vi "HFRR ADV v033 new software.vi"() -> ()   [LabVIEW 2025] (continued)
            n2885 = call <vilib>:"Read Characters From File.vi"("file path (dialog if empty)"=w3937, "start of read offset (chars.:0)"=60 ("start of read offset (chars.: 0)")) -> ("character string"=→"String Indicator 2":string)  [unwired: 4 in, 3 out]
          }
        }
        n2886 = call <vilib>:"Query Available Printers.vi"() -> ("system configured printers"=w3629:string[])  [unwired: 9 in, 2 out]
        "System Configured Printers 2" <- w3629
        n2887 = local read "OK Button 16"() -> (w3626:bool)
        n2888 = case shown="True" "OK Button 16" {
          frame False {
          }
          frame True {
            n2889 = stacked-sequence {
              frame #0 {
                n2890 = local read "Numeric 16"() -> (w3954:i32)
                n2891 = local write "Numeric 10"(w3954) -> ()
              }
              frame #1 {
                n2892 = local read "String 29"() -> (w3957:string)
                n2893 = String To Path(string=w3957) -> (path=w3956:path)
                n2894 = Open/Create/Replace File "Open File"(file path (use dialog)=w3956) -> (refnum out=w3958:refnum<file>)  [unwired: 5 in, 2 out]
                n2895 = for {
                  N: 16 -> [_]
                  tunnel: w3958 -> [w3965]
                  i -> [w3961]
                  (unwired) TRUE ("line mode (F)")
                  n2896 = Read from Text File "Read File"(file (use dialog)=w3965) -> (text=w3959:string)  [unwired: 3 in, 3 out]
                  n2897 = Match Pattern(string=w3959, regular expression="(") -> (after substring=w3964:string)  [unwired: 1 in, 3 out]
                  n2898 = Match Pattern(string=w3964, regular expression=")") -> (before substring=w3960:string)  [unwired: 1 in, 3 out]
                  n2899 = case shown="1" w3961 {
                    tunnel: w3960 -> [w3966 w3967 _ _ w3968 w3969 w3970 w3972 w3974 w3976 w3978 w3980 w3982 w3984 _]
                    tunnel: w3959 -> [_ _ _ _ _ _ _ _ _ _ _ _ _ _ _]
                    frame 0 {
                      "TITTLE" <- w3966
                    }
                    frame 1 {
                      "Sample ID" <- w3967
                    }
                    frame 2 {
                    }
                    frame 3 {
                    }
                    frame 4 {
                      "Test Date" <- w3968
                    }
                    frame 5 {
                      "Tested by" <- w3969
                    }
                    frame 6 {
                      n2900 = Fract/Exp String To Number(string=w3970) -> (number=→"Humidity before test 2":dbl)  [unwired: 3 in, 1 out]
                    }
                    frame 7 {
                      n2901 = Fract/Exp String To Number(string=w3972) -> (number=→"Temperature before test 2":dbl)  [unwired: 3 in, 1 out]
                    }
                    frame 8 {
                      n2902 = Fract/Exp String To Number(string=w3974) -> (number=→"Humidity after test 2":dbl)  [unwired: 3 in, 1 out]
                    }
                    frame 9 {
                      n2903 = Fract/Exp String To Number(string=w3976) -> (number=→"Temperature after test 2":dbl)  [unwired: 3 in, 1 out]
                    }
                    frame 10 {
                      n2904 = Fract/Exp String To Number(string=w3978) -> (number=→"MWSD 2":dbl)  [unwired: 3 in, 1 out]
                    }
                    frame 11 {
                      n2905 = Fract/Exp String To Number(string=w3980) -> (number=→"AVP 2":dbl)  [unwired: 3 in, 1 out]
                    }
                    frame 12 {
                      n2906 = Fract/Exp String To Number(string=w3982) -> (number=→"HCF 2":dbl)  [unwired: 3 in, 1 out]
                    }
                    frame 13 {
                      n2907 = Fract/Exp String To Number(string=w3984) -> (number=→"WS1.4 2":dbl)  [unwired: 3 in, 1 out]
                    }
                    frame 14, Default {
                    }
                  }
                }
              }
              frame #2 {
              }
            }
            n2908 = local write "OK Button 16"(FALSE ("OK Button 13")) -> ()
          }
        }
        n2909 = Index Array(array=w3629, index="Select Printer 3") -> (element=w3631:string)
        "Selected Printer" <- w3631
        n2910 = case shown="True" w3626 {
          frame False {
          }
          frame True {
            n2911 = flat-sequence {
              frame #0 {
              }
              frame #1 {
                n2912 = Wait (ms)(milliseconds to wait=u32 100) -> ()  [unwired: 1 out]
              }
              frame #2 {
                n2913 = local write "OK Button 16"(FALSE ("Print 3")) -> ()
              }
            }
          }
        }
        n2914 = case shown="True" "Print" {
          tunnel: w3631 -> [_ w3923]
          frame False {
          }
          frame True {
            (unwired) i16 6 ("width (-)")
            (unwired) "TESTED BY : "
            (unwired) "TESTED DATE :"
            (unwired) "SAMPLE ID : "
            (unwired) "SAMPLE DESIGN : "
            w3881 = "\r"
            w3898 = "\r"
            # "add image"
            n2915 = local read "Sample ID"() -> (w3871:string)
            n2916 = local read "Tested by"() -> (w3874:string)
            n2917 = local read "String 34"() -> (w3861:string)
            n2918 = local read "String 45"() -> (w3841:string)
            n2919 = local read "String 35"() -> (w3856:string)
            n2920 = local read "String 37"() -> (w3854:string)
            n2921 = local read "String 32"() -> (w3876:string)
            n2922 = local read "String 36"() -> (w3851:string)
            n2923 = local read "String 31"() -> (w3875:string)
            n2924 = local read "Test Date"() -> (w3872:string)
            n2925 = local read "String 33"() -> (w3877:string)
            n2926 = local read "String 38"() -> (w3847:string)
            n2927 = local read "String 39"() -> (w3844:string)
            n2928 = local write "Print"(FALSE ("Print FF")) -> ()
            n2929 = local read "S 39"() -> (w3859:string)
            n2930 = local read "S 38"() -> (w3866:string)
            n2931 = local read "Temperature before test 2"() -> (w3897:dbl)
            n2932 = local read "Temperature after test 2"() -> (w3887:dbl)
            n2933 = local read "Humidity before test 2"() -> (w3912:dbl)
            n2934 = local read "Humidity after test 2"() -> (w3896:dbl)
            n2935 = local read "MWSD 2"() -> (w3901:dbl)
            n2936 = local read "WS1.4 2"() -> (w3879:dbl)
            n2937 = Concatenate Strings("2)" ("string"), w3861) -> (w3862:string)
            n2938 = Concatenate Strings("3)" ("string"), w3859) -> (w3860:string)
            n2939 = Concatenate Strings("1)" ("string"), w3866) -> (w3865:string)
            n2940 = Concatenate Strings("4)" ("string"), w3856) -> (w3857:string)
            n2941 = Concatenate Strings("5)" ("string"), w3854) -> (w3853:string)
            n2942 = Concatenate Strings("6)" ("string"), w3851) -> (w3850:string)
            n2943 = Concatenate Strings("7)" ("string"), w3847) -> (w3848:string)
            n2944 = Concatenate Strings("8)" ("string"), w3844) -> (w3845:string)
            n2945 = local read "HCF 2"() -> (w3883:dbl)
            n2946 = local read "AVP 2"() -> (w3900:dbl)
            n2947 = local read "s.NO"() -> (w3842:string)
            n2948 = call <vilib>:"New Report.vi"("report type"=enum16{"Standard Report", "HTML"}."Standard Report") -> ("report out"=w3921:refnum<class "NI_report.lvclass">, "error out"=w3920:errorcluster)  [unwired: 13 in]
            n2949 = local read "TITTLE"() -> (w3873:string)
            n2950 = Concatenate Strings(w3898, w3841, w3842, w3898, w3876, w3871, w3898, w3875, w3872, w3898, w3877, w3874, w3898) -> (w3891:string)
            "test by" <- w3891
            n2951 = Number To Fractional String(number=w3897, width (-)=i16 6, precision (6)=i16 2) -> (F-format string=w3886:string)  [unwired: 1 in]
            n2952 = Number To Fractional String(number=w3896, width (-)=i16 6, precision (6)=i16 2) -> (F-format string=w3899:string)  [unwired: 1 in]
            n2953 = Number To Fractional String(number=w3912, width (-)=i16 6, precision (6)=i16 2) -> (F-format string=w3917:string)  [unwired: 1 in]
            n2954 = Number To Fractional String(number=w3901, width (-)=i16 6, precision (6)=i16 2) -> (F-format string=w3903:string)  [unwired: 1 in]
            n2955 = Number To Fractional String(number=w3887, width (-)=i16 6, precision (6)=i16 2) -> (F-format string=w3888:string)  [unwired: 1 in]
            n2956 = Number To Fractional String(number=w3900, width (-)=i16 6, precision (6)=i16 2) -> (F-format string=w3902:string)  [unwired: 1 in]
            n2957 = Number To Fractional String(number=w3883, width (-)=i16 6, precision (6)=i16 2) -> (F-format string=w3882:string)  [unwired: 1 in]
            n2958 = Number To Fractional String(number=w3879, precision (6)=i16 2) -> (F-format string=w3878:string)  [unwired: 2 in]
            n2959 = call-dynamic "Set Report Header Text.vi"("report in"=w3921, "center header text"=w3873, "error in (no error)"=w3920) -> ("report out"=w3892:refnum<class "NI_report.lvclass">, "error out"=w3893:errorcluster)  [unwired: 11 in]
            n2960 = Concatenate Strings(w3881, w3865, w3917, w3881, w3862, w3886, w3881, w3860, w3899, w3881, w3857, w3888, w3881, w3853, w3903, w3881, w3850, w3902, w3881, w3848, w3882, w3881, w3845, w3878) -> (w3869:string)
            "export 2" <- w3869
            n2961 = call-poly <vilib>:"Append Report Text.vi"("report in"=w3892, "text"=w3891, "error in (no error)"=w3893) -> ("report out"=w3895:refnum<class "NI_report.lvclass">, "error out"=w3894:errorcluster)  [unwired: 9 in, 2 out]
            n2962 = local read "test by"() -> (w3868:string)
            n2963 = local read "TITTLE"() -> (w3870:string)
            n2964 = call-poly <vilib>:"Append Report Text.vi"("report in"=w3895, "error in (no error)"=w3894) -> ("report out"=w3916:refnum<class "NI_report.lvclass">, "error out"=w3914:errorcluster)  [unwired: 10 in, 2 out]
            n2965 = Concatenate Strings(w3870, w3869, w3868) -> (→"output":string)
            n2966 = call-poly <vilib>:"Append Report Text.vi"("report in"=w3916, "text"=w3869, "error in (no error)"=w3914) -> ("report out"=w3915:refnum<class "NI_report.lvclass">, "error out"=w3913:errorcluster)  [unwired: 9 in, 2 out]
            n2967 = call-dynamic "Print Report.vi"("report in"=w3915, "printer name (default)"=w3923, "error in (no error)"=w3913) -> ("report out"=w3925:refnum<class "NI_report.lvclass">, "error out"=w3926:errorcluster)  [unwired: 11 in]
            n2968 = call-dynamic "Dispose Report.vi"("report in"=w3925, "error in (no error)"=w3926) -> ()  [unwired: 13 in, 1 out]
          }
        }
        n2969 = case shown="True" "Print 2" {
          frame False {
          }
          frame True {
            n2970 = flat-sequence {
              frame #0 {
                n2971 = local read "s.NO"() -> (→"s.NO 2":string)
                n2972 = Wait (ms)(milliseconds to wait=u32 20) -> ()  [unwired: 1 out]
                n2973 = local read "Sample ID  3"() -> (→"Sample ID  6":string)
                n2974 = local read "Sample ID  4"() -> (→"Sample ID  7":string)
                n2975 = local read "Sample ID"() -> (→"Sample ID  2":string)
                n2976 = local read "Tested by"() -> (→"Tested by 2":string)
                n2977 = local read "Test Date"() -> (→"Test Date 2":string)
                n2978 = local read "Humidity after test 3"() -> (→"Humidity after test 4":dbl)
                n2979 = local read "Ref A Test Date :"() -> (→"TITTLE 4":string)
                n2980 = local read "Temperature before test 3"() -> (w3748:dbl)
                n2981 = local read "Temperature before test 3"() -> (→"Temperature after test 5":dbl)
                n2982 = local read "Temperature after test 3"() -> (→"Temperature after test 4":dbl)
                n2983 = local read "Humidity before test 3"() -> (→"Humidity before test 4":dbl)
                n2984 = local write "Temperature before test 3"(w3748) -> ()
                n2985 = local read "image data"() -> (w3739:T16)
                n2986 = String To Path(string="C:\\LAB-IQ\\im\\Temp_resized.jpg") -> (path=w3740:path)
                "path 2" <- w3740
                n2987 = call <vilib>:"Write JPEG File.vi"("image data"=w3739, "path to JPEG file"=w3740) -> ()  [unwired: 8 in, 2 out]
                "Ref A Test Date :" <- "Ref A Test Date :"
                "Ref B Test Date :" <- "Ref B Test Date :"
                "Ref B Scar Value :" <- "Ref B Scar Value :"
                "Ref A Scar Value :" <- "Ref A Scar Value :"
              }
              frame #1 {
                (unwired) HTML_Report_Image_Alignment."MIDDLE" ("alignment (default)")
                w3776 = u16 0 items=["portrait", "landscape"] ("orientation (portrait)")
                (unwired) HTML_Report_Image_Alignment."ABSMIDDLE" ("alignment (default)")
                (unwired) "TESTED BY : "
                (unwired) "TESTED DATE :"
                (unwired) "SAMPLE ID : "
                (unwired) "SAMPLE DESIGN : "
                w3809 = "\r"
                # "add image"
                n2988 = Wait (ms)(milliseconds to wait=u32 20) -> ()  [unwired: 1 out]
                n2989 = local read "Sample ID  2"() -> (w3802:string)
                n2990 = local read "Wear Scar X"() -> (w3774:dbl)
                "Length ( microns ) 2" <- w3774
                n2991 = local read "Wear Scar Y"() -> (w3773:dbl)
                "Wear Scar Y ( microns ) :" <- w3773
                n2992 = local read "Test Date 2"() -> (w3803:string)
                n2993 = local read "Tested by 2"() -> (w3804:string)
                n2994 = local read "String 46"() -> (w3800:string)
                n2995 = local read "String 48"() -> (w3806:string)
                n2996 = local read "String 47"() -> (w3805:string)
                n2997 = local read "String 49"() -> (w3807:string)
                n2998 = local read "String 10"() -> (w3760:string)
                n2999 = local read "s.NO 2"() -> (w3801:string)
                n3000 = Add(x=w3774, y=w3773) -> (x+y=w3772:dbl)
                n3001 = call <vilib>:"New Report.vi"("report type"=enum16{"Standard Report", "HTML"}."HTML") -> ("report out"=w3780:refnum<class "NI_report.lvclass">, "error out"=w3778:errorcluster)  [unwired: 13 in]
                n3002 = Concatenate Strings(w3809, w3800, w3801, w3809, w3806, w3802, w3809, w3805, w3803, w3809, w3807, w3804, w3809) -> (→"test by 2":string)
                n3003 = Concatenate Strings("C:\\LAB-IQ\\Data\\" ("string"), w3760, ".jpg" ("string")) -> ()  [unwired: 1 out]
                n3004 = Divide(x=w3772, y=2.0) -> (x/y=→"Mean Wear ( microns) :":dbl)
                n3005 = call-dynamic "Set Report Orientation.vi"("report in"=w3780, "orientation (portrait)"=w3776, "error in (no error)"=w3778) -> ("report out"=w3779:refnum<class "NI_report.lvclass">, "error out"=w3777:errorcluster)  [unwired: 11 in]
                n3006 = for {
                  N: 5 -> [_]
                  tunnel: w3779 -> [w3830]
                  tunnel: [w3829] -> w3758
                  tunnel: w3777 -> [w3828]
                  tunnel: [w3827] -> w3757
                  n3007 = call-dynamic "Set Report Tab Width.vi"("report in"=w3830, "error in (no error)"=w3828) -> ("report out"=w3829:refnum<class "NI_report.lvclass">, "error out"=w3827:errorcluster)  [unwired: 12 in]
                }
                n3008 = local read "TITTLE"() -> (w3775:string)
                n3009 = call-dynamic "Set Report Header Text.vi"("report in"=w3758, "center header text"=w3775, "error in (no error)"=w3757) -> ("report out"=w3796:refnum<class "NI_report.lvclass">, "error out"=w3795:errorcluster)  [unwired: 11 in]
                n3010 = for {
                  N: 1 -> [_]
                  tunnel: [w3834] -> w3782
                  tunnel: [w3833] -> w3781
                  tunnel: w3796 -> [w3832]
                  tunnel: w3795 -> [w3831]
                  n3011 = call-dynamic "New Report Line.vi"("report in"=w3832, "error in (no error)"=w3831) -> ("report out"=w3834:refnum<class "NI_report.lvclass">, "error out"=w3833:errorcluster)  [unwired: 12 in]
                }
                n3012 = for {
                  N: 2 -> [_]
                  tunnel: [w3826] -> w3788
                  tunnel: [w3825] -> w3787
                  tunnel: w3782 -> [w3824]
                  tunnel: w3781 -> [w3823]
                  n3013 = call-dynamic "New Report Line.vi"("report in"=w3824, "error in (no error)"=w3823) -> ("report out"=w3826:refnum<class "NI_report.lvclass">, "error out"=w3825:errorcluster)  [unwired: 12 in]
                }
                n3014 = for {
                  N: 25 -> [_]
                  tunnel: w3788 -> [w3822]
                  tunnel: w3787 -> [w3820]
                  tunnel: [w3821] -> w3791
                  tunnel: [w3819] -> w3790
                  n3015 = call-dynamic "Set Report Tab Width.vi"("report in"=w3822, "error in (no error)"=w3820) -> ("report out"=w3821:refnum<class "NI_report.lvclass">, "error out"=w3819:errorcluster)  [unwired: 12 in]
                }
                n3016 = control-ref of="Tab Control 9"() -> (w3786:refnum<vi>)
                n3017 = call-dynamic "Append Control Image to Report.vi"("report in"=w3791, "alignment (default)"=HTML_Report_Image_Alignment."ABSMIDDLE", "ctrl reference"=w3786, "error in (no error)"=w3790) -> ("report out"=w3785:refnum<class "NI_report.lvclass">, "error out"=w3784:errorcluster)  [unwired: 8 in, 2 out]
                n3018 = for {
                  N: 3 -> [_]
                  tunnel: [w3818] -> w3769
                  tunnel: [w3817] -> w3768
                  tunnel: w3785 -> [w3816]
                  tunnel: w3784 -> [w3815]
                  n3019 = call-dynamic "New Report Line.vi"("report in"=w3816, "error in (no error)"=w3815) -> ("report out"=w3818:refnum<class "NI_report.lvclass">, "error out"=w3817:errorcluster)  [unwired: 12 in]
                }
                n3020 = for {
                  N: 100 -> [_]
                  tunnel: w3769 -> [w3814]
                  tunnel: w3768 -> [w3812]
                  tunnel: [w3813] -> w3765
                  tunnel: [w3811] -> w3763
                  n3021 = call-dynamic "Set Report Tab Width.vi"("report in"=w3814, "error in (no error)"=w3812) -> ("report out"=w3813:refnum<class "NI_report.lvclass">, "error out"=w3811:errorcluster)  [unwired: 12 in]
                }
                n3022 = String To Path(string="C:\\LAB-IQ\\im\\Temp_resized.jpg") -> (path=w3755:path)
                n3023 = call-poly <vilib>:"Append Image to Report.vi"("report in"=w3765, "path or URL of image"=w3755, "error in (no error)"=w3763) -> ("report out"=w3764:refnum<class "NI_report.lvclass">, "error out"=w3762:errorcluster)  [unwired: 9 in, 2 out]
                n3024 = call-poly <vilib>:"Open HTML Report in Browser.vi"("report in"=w3764, "error in (no error)"=w3762) -> ("report out"=w3799:refnum<class "NI_report.lvclass">, "error out"=w3798:errorcluster)  [unwired: 11 in, 1 out]
                n3025 = call-dynamic "Dispose Report.vi"("report in"=w3799, "error in (no error)"=w3798) -> ()  [unwired: 13 in, 1 out]
              }
              frame #2 {
              }
              frame #3 {
                n3026 = disable-structure shown="Disabled" {
                  frame Disabled {
                    n3027 = local read "String 10"() -> (w3839:string)
                    n3028 = Concatenate Strings("C:\\LAB-IQ-NXT\\Data\\" ("string"), w3839, ".jpg" ("string")) -> (w3837:string)
                    n3029 = String To Path(string=w3837) -> (path=w3836:path)
                    n3030 = Delete(path (use dialog)=w3836) -> ()  [unwired: 4 in, 3 out]
                  }
                  frame Enabled {
                  }
                }
                n3031 = local write "Print 2"(FALSE ("Print")) -> ()
              }
            }
          }
        }
      }
    }
    n3032 = Wait (ms)(milliseconds to wait=u32 50) -> ()  [unwired: 1 out]
    n3033 = Wait (ms)(milliseconds to wait=u32 50) -> ()  [unwired: 1 out]
    n3034 = local read "Quit"() -> (w2175:bool)
  }
  n3035 = VISA Close(VISA resource name=w41, error in (no error)=w40) -> ()  [unwired: 1 out]
  n3036 = while {
    stop <- w3990 stop-if-true
    n3037 = local read "Auto Start Test"() -> (w3988:bool)
    n3038 = local read "RUN"() -> (w3987:bool)
    n3039 = Wait (ms)(milliseconds to wait=u32 1000) -> ()  [unwired: 1 out]
    n3040 = Or(x=w3987, y=w3988) -> (x .or. y?=w3986:bool)
    n3041 = case shown="True" w3986 {
      frame False {
      }
      frame True {
        n3042 = local read "LVDT STROKE Actual"() -> (w3991:dbl)
        n3043 = In Range and Coerce(upper limit=1.2, x=w3991, lower limit=0.6) -> (In Range?=w3994:bool)  [unwired: 1 out]
        n3044 = call-poly <vilib>:"Random Number (Range).vi"("lower bound (0)"=0.998 ("upper bound (100)"), "upper bound (100)"=1.003) -> ("number"=w3992:dbl)  [unwired: 9 in]
        n3045 = case shown="True" w3994 {
          tunnel: [w3999 w4000] -> w3993
          tunnel: w3992 -> [_ w4000]
          tunnel: w3991 -> [w3999 _]
          frame False {
          }
          frame True {
          }
        }
        "LVDT STROKE DISPLAY" <- w3993
      }
    }
    n3046 = local read "Quit"() -> (w3990:bool)
  }
  n3047 = while {
    tunnel: [w4017] -> w49
    shift-right: [w4010] -> _
    shift-left: 0.0 -> [w4013]
    shift-right: [w4009] -> _
    shift-left: 0.0 -> [w4012]
    shift-right: [w4008] -> _
    shift-left: 100.0 ("vc_cmd") -> [w4011]
    stop <- w4017 stop-if-true
    # "PID LOGIC"
    n3048 = local read "run test Calibration"() -> (w4005:bool)
    n3049 = local read "RUN"() -> (w4015:bool)
    n3050 = local read "Auto Start Temp"() -> (w4006:bool)
    n3051 = local read "Auto Start Test"() -> (w4014:bool)
    n3052 = local read "START TEMP"() -> (w4004:bool)
    n3053 = And(x=w4006, y=w4014) -> (x .and. y?=w4007:bool)
    n3054 = Or(x=w4015, y=w4007) -> (x .or. y?=w4016:bool)
    n3055 = And(x=w4016, y=w4004) -> (x .and. y?=w4003:bool)
    n3056 = And(x=w4005, y=w4004) -> (x .and. y?=w4002:bool)
    n3057 = Or(x=w4002, y=w4003) -> (x .or. y?=w4001:bool)
    n3058 = Wait (ms)(milliseconds to wait="milliseconds to wait") -> ()  [unwired: 1 out]
    n3059 = case shown="True" w4001 {
      tunnel: [400.0 ("out_vc_cmd") w4036] -> w4008
      tunnel: [w4020 w4038] -> w4009
      tunnel: [w4020 w4037] -> w4010
      tunnel: w4013 -> [_ w4027]
      tunnel: w4012 -> [_ w4026]
      tunnel: w4011 -> [_ w4025]
      tunnel: w4005 -> [_ w4021]
      frame False {
        w4020 = 0.0 ("error_out")
      }
      frame True {
        n3060 = case shown="True" w4021 {
          tunnel: [w4045 1.0] -> w4023
          frame False {
            n3061 = local read "Set Strk"() -> (w4044:dbl)
            n3062 = Add(x=w4044, y="Add up Stroke") -> (x+y=w4045:dbl)
          }
          frame True {
          }
        }
        n3063 = local read "LVDT STROKE"() -> (w4022:dbl)
        n3064 = formula code="// Zero-Hardcode Explicit Positional-Form PID Engine\n// Inputs: target_stroke, measured_stroke, dt, prev_error, integral_accumulator_in, prev_vc_cmd\n//         kp, ki, kd, max_step_change, max_amplitude, min_amplitude, startup_cmd\n// Outputs: vc_cmd, error_out, out_error, integral_accumulator_out, out_vc_cmd\n\n// 1. Calculate Tracking Error\nfloat current_error = target_stroke - measured_stroke;\nerror_out = current_error;\n\n// 2. Compute Proportional Term\nfloat p_term = kp * current_error;\n\n// 3. Compute Derivative Term\nfloat d_term = 0.0;\nif (dt > 0.0) {\n    d_term = kd * ((current_error - prev_error) / dt);\n}\n\n// 4. Update and Accumulate Integral Term\nfloat current_integral = integral_accumulator_in + (current_error * dt);\nfloat i_term = ki * current_integral;\n\n// 5. Calculate Ideal Target Command (Anchored by startup baseline)\nfloat ideal_command = startup_cmd + p_term + i_term + d_term;\n\n// 6. Apply Loop Rate Limiting FIRST \n// (Forces the command to climb gradually from prev_vc_cmd instead of jumping straight to max)\nfloat raw_adjustment = ideal_command - prev_vc_cmd;\n\nif (raw_adjustment > max_step_change) {\n    raw_adjustment = max_step_change;\n} else if (raw_adjustment < -max_step_change) {\n    raw_adjustment = -max_step_change;\n}\n\nfloat next_vc_cmd = prev_vc_cmd + raw_adjustment;\n\n// 7. Anti-Windup Protection & Final Output Safety Safeguard Clamping\n// (Back-calculating based on what we are ACTUALLY outputting)\nif (next_vc_cmd > max_amplitude) {\n    float excess = next_vc_cmd - max_amplitude;\n    if (ki > 0.0) {\n        current_integral -= excess / ki;\n    }\n    next_vc_cmd = max_amplitude;\n} else if (next_vc_cmd < min_amplitude) {\n    float excess = next_vc_cmd - min_amplitude;\n    if (ki > 0.0) {\n        current_integral -= excess / ki;\n    }\n    next_vc_cmd = min_amplitude;\n}\n\n// 8. Map to Shift Registers for memory persistence\nvc_cmd = next_vc_cmd;\nout_error = current_error;                   \nintegral_accumulator_out = current_integral;  \nout_vc_cmd = next_vc_cmd;"("target_stroke"=w4023, "measured_stroke"=w4022, "dt"="dt", "integral_accumulator_in"=w4026, "prev_error"=w4027, "prev_vc_cmd"=w4025, "kp"="kp", "ki"="ki", "kd"="kd", "max_step_change"="max_step_change", "max_amplitude"="max_amplitude", "min_amplitude"="min_amplitude", "startup_cmd"="startup_cmd") -> ("vc_cmd"=w4042:dbl, "out_error"=w4037:dbl, "integral_accumulator_out"=w4038:dbl, "out_vc_cmd"=w4036:dbl)  [unwired: 1 out]
        "output Vpp" <- w4042
        n3065 = Number To Fractional String(number=w4042, precision (6)=i16 1) -> (F-format string=w4040:string)  [unwired: 2 in]
        n3066 = Concatenate Strings("DAC;" ("string"), w4040) -> (w4024:string)
        n3067 = local write "Due Write"(w4024) -> ()
        "prev_error" <- w4027
        "integral_accumulator_in" <- w4026
        "prev_vc_cmd" <- w4025
      }
    }
    n3068 = local read "Quit"() -> (w4017:bool)
  }
  n3069 = Or(x=w45, y=w44) -> (x .or. y?=w46:bool)
  n3070 = Or(x=w42, y=w46) -> (x .or. y?=w51:bool)
  n3071 = control-ref of="new picture"() -> ()  [unwired: 1 out]
  n3072 = Or(x=w54, y=w51) -> (x .or. y?=w48:bool)
  n3073 = Or(x=w48, y=w49) -> (x .or. y?=w43:bool)
  n3074 = while {
    tunnel: [w4047] -> w53
    i -> [w4054]
    stop <- w4047 stop-if-true
    n3075 = local read "Quit"() -> (w4047:bool)
    n3076 = Equal To 0?(x=w4054) -> (x = 0?=w4052:bool)
    n3077 = call "Elapsed Time3"("Time Target (s)"=45.0, "Auto Reset"=TRUE) -> ("Time has Elapsed"=w4051:bool)  [unwired: 10 in, 7 out]
    n3078 = Wait (ms)(milliseconds to wait=u32 50) -> ()  [unwired: 1 out]
    n3079 = Or(x=w4051, y=w4052) -> (x .or. y?=w4053:bool)
    n3080 = case shown="True" w4053 {
      frame False {
      }
      frame True {
        n3081 = call <vilib>:"System Exec.vi"("run minimized? (F)"=TRUE, "error in (no error)"="error in (no error)", "command line"="powercfg.exe -change -monitor-timeout-ac 0") -> ("error out"=w4065:errorcluster)  [unwired: 5 in, 3 out]
        n3082 = call <vilib>:"System Exec.vi"("run minimized? (F)"=TRUE, "error in (no error)"=w4065, "command line"="powercfg.exe -change -disk-timeout-ac 0") -> ("error out"=w4064:errorcluster)  [unwired: 5 in, 3 out]
        n3083 = call <vilib>:"System Exec.vi"("run minimized? (F)"=TRUE, "error in (no error)"=w4064, "command line"="powercfg.exe -change -standby-timeout-ac 0") -> ("error out"=w4063:errorcluster)  [unwired: 5 in, 3 out]
        n3084 = call <vilib>:"System Exec.vi"("run minimized? (F)"=TRUE, "error in (no error)"=w4063, "command line"="powercfg.exe -change -hibernate-timeout-ac 0") -> ("error out"=w4062:errorcluster)  [unwired: 5 in, 3 out]
        n3085 = call <vilib>:"Simple Error Handler.vi"("error in (no error)"=w4062) -> ("error out"=w4068:errorcluster)  [unwired: 4 in, 4 out]
        n3086 = call <vilib>:"Clear Errors.vi"("error in (no error)"=w4068) -> ("error out"=→"error out":errorcluster)  [unwired: 5 in, 1 out]
      }
    }
  }
  n3087 = Compound Arithmetic op=OR(w56, w43, w53) -> (w55:bool)
  n3088 = flat-sequence {
    tunnel: w55 -> [_]
    tunnel: [w4070] -> w25
    tunnel: w25 -> [_]
    frame #0 {
      n3089 = call "CLOSE CONNECTION.vi"() -> ("error out"=w4070:errorcluster)  [unwired: 11 in]
    }
    frame #1 {
      n3090 = Quit LabVIEW(quit? (T)=TRUE) -> ()
      n3091 = local write "Quit"(FALSE ("EXIT")) -> ()
    }
  }
  n3092 = property on="Heater Button" class="Bool (strict)"("Visible"=TRUE) -> ()  [unwired: 2 in, 2 out]
  n3093 = while {
    tunnel: [w4077] -> _
    i -> [w4077]
    stop <- w4073 stop-if-true
    # "Langauage selection"
    n3094 = Equal?(x="Lan flag", y=22.0) -> ()  [unwired: 1 out]
    n3095 = disable-structure shown="Disabled" {
      frame Disabled {
        n3096 = stacked-sequence {
          frame #0 {
            n3097 = case shown="\"Russian\"" "Language Selection" {
              tunnel: [0 1] -> w4079
              frame "English", Default {
              }
              frame "Russian" {
              }
            }
            n3098 = for {
              N: 130 -> [_]
              tunnel: "Table" -> [w4088]
              tunnel: w4079 -> [w4087]
              i -> [w4086]
              n3099 = Index Array(array=w4088, index (row)=w4086, index (col)=w4087) -> (element=w4085:string)
              n3100 = case shown="1" w4086 {
                tunnel: w4085 -> [w4089 w4090 _ w4091 w4092 w4093 w4094 w4095 w4096 w4097 w4098 w4099 w4100 w4101 w4102 w4103 w4104 w4105 w4106 w4107 w4108 w4109 w4110 w4111 w4112 w4113 w4114 w4115 w4116 _ _ w4117 w4118 w4119 w4120 w4121 w4122 w4131 w4138 w4145 w4152 w4156 w4159 w4162 w4164 w4166 w4167 w4168 w4169 w4170 w4171 w4172 w4173 w4174 w4175 w4176 w4177 w4178 w4179 w4180 w4181 w4182 w4183 w4184 w4185 w4186 w4187 w4188 w4189 w4190 w4191 w4192 w4193 w4194 w4195 w4196 w4197 w4198 w4199 w4200 w4201 w4202 w4203 w4204 w4205 w4206 w4207 w4208 w4209 w4210 w4211 w4212 w4213 w4214 w4215 w4216 w4217 w4218 w4219 w4220 w4221 w4222 w4223 w4224 w4225 _ w4226 w4227 w4228 w4229 w4230 w4231 w4232 w4233 w4234 w4235 w4236 w4237 w4238 _ w4239 w4240 w4241 w4242 w4243 w4244 _]
                frame 0 {
                  n3101 = local write "S"(w4089) -> ()
                }
                frame 1 {
                  n3102 = local write "S 2"(w4090) -> ()
                }
                frame 2 {
                }
                frame 3 {
                  n3103 = local write "S 4"(w4091) -> ()
                }
                frame 4 {
                  n3104 = property on="FILE" class="Str"("Caption.Text"=w4092) -> ()  [unwired: 2 in, 2 out]
                }
                frame 5 {
                  n3105 = property on="Fuel Discription :" class="Str"("Caption.Text"=w4093) -> ()  [unwired: 2 in, 2 out]
                }
                frame 6 {
                  n3106 = property on="Remarks :" class="Str"("Caption.Text"=w4094) -> ()  [unwired: 2 in, 2 out]
                }
                frame 7 {
                  n3107 = property on="Save & Continue" class="Bool (strict)"("Boolean Text.Text"=w4095) -> ()  [unwired: 2 in, 2 out]
                }
                frame 8 {
                }
                frame 9 {
                  n3108 = property on="Set Hz" class="DigNum (strict)"("Caption.Text"=w4097) -> ()  [unwired: 2 in, 2 out]
                }
                frame 10 {
                }
                frame 11 {
                  n3109 = property on="NORMAL LOAD" class="DigNum (strict)"("Caption.Text"=w4099) -> ()  [unwired: 2 in, 2 out]
                }
                frame 12 {
                }
                frame 13 {
                  n3110 = property on="Set Temp" class="DigNum (strict)"("Caption.Text"=w4101) -> ()  [unwired: 2 in, 2 out]
                }
                frame 14 {
                  n3111 = local write "S 15"(w4102) -> ()
                }
                frame 15 {
                  n3112 = property on="Set Rh" class="DigNum (strict)"("Caption.Text"=w4103) -> ()  [unwired: 2 in, 2 out]
                }
                frame 16 {
                }
                frame 17 {
                  n3113 = local write "S 18"(w4105) -> ()
                }
                frame 18 {
                  "String 17" <- w4106
                }
                frame 19 {
                  n3114 = property on="test time" class="DigNum (strict)"("Caption.Text"=w4107) -> ()  [unwired: 2 in, 2 out]
                }
                frame 20 {
                  "String 18" <- w4108
                  "String 22" <- w4108
                }
                frame 21 {
                  n3115 = property on="Elapsed time" class="DigNum (strict)"("Caption.Text"=w4109) -> ()  [unwired: 2 in, 2 out]
                }
                frame 22 {
                  n3116 = property on="Samplingtime 2" class="DigNum (strict)"("Caption.Text"=w4110) -> ()  [unwired: 2 in, 2 out]
                }
                frame 23 {
                  "String 21" <- w4111
                }
                frame 24 {
                  n3117 = property on="Countdown" class="DigNum (strict)"("Caption.Text"=w4112) -> ()  [unwired: 2 in, 2 out]
                }
                frame 25 {
                  n3118 = property on="Countdown 2" class="DigNum (strict)"("Caption.Text"=w4113) -> ()  [unwired: 2 in, 2 out]
                }
                frame 26 {
                  n3119 = property on="Engage" class="Bool (strict)"("Boolean Text.Text"=w4114) -> ()  [unwired: 2 in, 2 out]
                }
                frame 27 {
                  n3120 = property on="Boolean  4" class="Bool (strict)"("Boolean Text.Text"=w4115) -> ()  [unwired: 2 in, 2 out]
                }
                frame 28 {
                  n3121 = property on="Test \nStatus" class="Bool (strict)"("Boolean Text.Text"=w4116) -> ()  [unwired: 2 in, 2 out]
                }
                frame 29 {
                }
                frame 30 {
                }
                frame 31 {
                }
                frame 32 {
                  n3122 = property on="RSTCOF" class="Bool"("Boolean Text.Text"=w4118) -> ()  [unwired: 2 in, 2 out]
                  n3123 = property on="RST FF" class="Bool"("Boolean Text.Text"=w4118) -> ()  [unwired: 2 in, 2 out]
                  n3124 = property on="RST TEMP" class="Bool"("Boolean Text.Text"=w4118) -> ()  [unwired: 2 in, 2 out]
                  n3125 = property on="RSTV1 3" class="Bool"("Boolean Text.Text"=w4118) -> ()  [unwired: 2 in, 2 out]
                  n3126 = property on="rstv2" class="Bool"("Boolean Text.Text"=w4118) -> ()  [unwired: 2 in, 2 out]
                  n3127 = property on="RSTV1 2" class="Bool"("Boolean Text.Text"=w4118) -> ()  [unwired: 2 in, 2 out]
                  n3128 = property on="RST CP" class="Bool"("Boolean Text.Text"=w4118) -> ()  [unwired: 2 in, 2 out]
                }
                frame 33 {
                  "S 61" <- w4119
                }
                frame 34 {
                  "String 23" <- w4120
                }
                frame 35 {
                  n3129 = property on="Rh Before" class="DigNum (strict)"("Caption.Text"=w4121) -> ()  [unwired: 2 in, 2 out]
                }
                frame 36 {
                  n3130 = Match Pattern(string=w4122, regular expression=",") -> (before substring=→"bs":string, after substring=→"as":string)  [unwired: 1 in, 2 out]
                  n3131 = property on="Rh After" class="DigNum (strict)"("Caption.Text"=w4122) -> ()  [unwired: 2 in, 2 out]
                }
                frame 37 {
                  n3132 = Match Pattern(string=w4131, regular expression=",") -> (before substring=w4130:string, after substring=w4129:string)  [unwired: 1 in, 2 out]
                  "bs" <- w4130
                  "as" <- w4129
                  n3133 = Concatenate Strings(w4130, w4129) -> (w4126:string)
                  n3134 = property on="Humidity before test 2" class="DigNum (strict)"("Caption.Text"=w4126) -> ()  [unwired: 2 in, 2 out]
                  n3135 = Concatenate Strings(w4126, "=" ("string")) -> (w4127:string)
                  n3136 = local write "S 38"(w4127) -> ()
                }
                frame 38 {
                  n3137 = Match Pattern(string=w4138, regular expression=",") -> (before substring=w4137:string, after substring=w4136:string)  [unwired: 1 in, 2 out]
                  "bs" <- w4137
                  "as" <- w4136
                  n3138 = Concatenate Strings(w4137, w4136) -> (w4133:string)
                  n3139 = property on="Humidity after test 2" class="DigNum (strict)"("Caption.Text"=w4133) -> ()  [unwired: 2 in, 2 out]
                  n3140 = Concatenate Strings(w4133, "=" ("string")) -> (w4135:string)
                  n3141 = local write "S 39"(w4135) -> ()
                }
                frame 39 {
                  n3142 = Match Pattern(string=w4145, regular expression=",") -> (before substring=w4144:string, after substring=w4143:string)  [unwired: 1 in, 2 out]
                  "bs" <- w4144
                  "as" <- w4143
                  n3143 = Concatenate Strings(w4144, w4143) -> (w4140:string)
                  n3144 = property on="Temperature before test 2" class="DigNum (strict)"("Caption.Text"=w4140) -> ()  [unwired: 2 in, 2 out]
                  n3145 = Concatenate Strings(w4140, "=" ("string")) -> (→"String 34":string)
                }
                frame 40 {
                  n3146 = Match Pattern(string=w4152, regular expression=",") -> (before substring=w4151:string, after substring=w4150:string)  [unwired: 1 in, 2 out]
                  "bs" <- w4151
                  "as" <- w4150
                  n3147 = Concatenate Strings(w4151, w4150) -> (w4147:string)
                  n3148 = property on="Temperature after test 2" class="DigNum (strict)"("Caption.Text"=w4147) -> ()  [unwired: 2 in, 2 out]
                  n3149 = Concatenate Strings(w4147, "=" ("string")) -> (→"String 35":string)
                  n3150 = property on="Temperature after test" class="DigNum (strict)"("Caption.Text"=w4147) -> ()  [unwired: 2 in, 2 out]
                }
                frame 41 {
                  n3151 = property on="AVP 2" class="DigNum (strict)"("Caption.Text"=w4156) -> ()  [unwired: 2 in, 2 out]
                  n3152 = Concatenate Strings(w4156, "=" ("string")) -> (→"String 36":string)
                }
                frame 42 {
                  n3153 = property on="MWSD 2" class="DigNum (strict)"("Caption.Text"=w4159) -> ()  [unwired: 2 in, 2 out]
                  n3154 = Concatenate Strings(w4159, "=" ("string")) -> (→"String 37":string)
                }
                frame 43 {
                  n3155 = property on="HCF 2" class="DigNum (strict)"("Caption.Text"=w4162) -> ()  [unwired: 2 in, 2 out]
                  n3156 = Concatenate Strings(w4162, "=" ("string")) -> (→"String 38":string)
                }
                frame 44 {
                  n3157 = Concatenate Strings(w4164, "=" ("string")) -> (→"String 39":string)
                  n3158 = property on="WS1.4 2" class="DigNum (strict)"("Caption.Text"=w4164) -> ()  [unwired: 2 in, 2 out]
                }
                frame 45 {
                }
                frame 46 {
                  n3159 = local write "S 47"(w4167) -> ()
                }
                frame 47 {
                  n3160 = local write "S 48"(w4168) -> ()
                }
                frame 48 {
                  n3161 = local write "S 49"(w4169) -> ()
                }
                frame 49 {
                  n3162 = local write "S 50"(w4170) -> ()
                }
                frame 50 {
                  n3163 = local write "S 51"(w4171) -> ()
                }
                frame 51 {
                  n3164 = local write "S 52"(w4172) -> ()
                }
                frame 52 {
                  n3165 = local write "S 53"(w4173) -> ()
                }
                frame 53 {
                  n3166 = local write "S 54"(w4174) -> ()
                }
                frame 54 {
                  n3167 = local write "S 55"(w4175) -> ()
                }
                frame 55 {
                  n3168 = local write "S 56"(w4176) -> ()
                }
                frame 56 {
                  n3169 = local write "S 57"(w4177) -> ()
                }
                frame 57 {
                  n3170 = local write "S 58"(w4178) -> ()
                }
                frame 58 {
                  n3171 = local write "S 59"(w4179) -> ()
                }
                frame 59 {
                  n3172 = local write "S 60"(w4180) -> ()
                }
                frame 60 {
                  n3173 = local write "S 62"(w4181) -> ()
                }
                frame 61 {
                  n3174 = local write "S 63"(w4182) -> ()
                }
                frame 62 {
                  n3175 = local write "S 64"(w4183) -> ()
                }
                frame 63 {
                  n3176 = local write "S 65"(w4184) -> ()
                }
                frame 64 {
                  n3177 = local write "S 66"(w4185) -> ()
                }
                frame 65 {
                  n3178 = local write "S 67"(w4186) -> ()
                }
                frame 66 {
                  n3179 = local write "S 68"(w4187) -> ()
                }
                frame 67 {
                  n3180 = local write "S 69"(w4188) -> ()
                }
                frame 68 {
                  n3181 = local write "S 70"(w4189) -> ()
                }
                frame 69 {
                  n3182 = local write "S 71"(w4190) -> ()
                }
                frame 70 {
                  n3183 = local write "S 72"(w4191) -> ()
                }
                frame 71 {
                  n3184 = local write "S 73"(w4192) -> ()
                }
                frame 72 {
                  n3185 = local write "S 74"(w4193) -> ()
                }
                frame 73 {
                  n3186 = local write "S 75"(w4194) -> ()
                }
                frame 74 {
                  n3187 = local write "S 76"(w4195) -> ()
                }
                frame 75 {
                  n3188 = local write "S 77"(w4196) -> ()
                }
                frame 76 {
                  n3189 = local write "S 78"(w4197) -> ()
                }
                frame 77 {
                  n3190 = local write "S 79"(w4198) -> ()
                }
                frame 79 {
                  n3191 = property on="Sample Temperature ( °C )" class="XYGraph (strict)"("Y Scale.Name Label.Text"=w4199) -> ()  [unwired: 2 in, 2 out]
                }
                frame 80 {
                  n3192 = local write "S 81"(w4200) -> ()
                  n3193 = property on="Humidity ( %RH )" class="XYGraph (strict)"("Y Scale.Name Label.Text"=w4200) -> ()  [unwired: 2 in, 2 out]
                }
                frame 78 {
                  n3194 = property on="Air Temperature  ( °C )" class="XYGraph (strict)"("X Scale.Name Label.Text"=w4201) -> ()  [unwired: 2 in, 2 out]
                  n3195 = property on="Humidity ( %RH )" class="XYGraph (strict)"("X Scale.Name Label.Text"=w4201) -> ()  [unwired: 2 in, 2 out]
                  n3196 = property on="Sample Temperature ( °C )" class="XYGraph (strict)"("X Scale.Name Label.Text"=w4201) -> ()  [unwired: 2 in, 2 out]
                  n3197 = property on="Coefficient Of Friction" class="XYGraph (strict)"("X Scale.Name Label.Text"=w4201) -> ()  [unwired: 2 in, 2 out]
                }
                frame 81 {
                  n3198 = property on="Air Temperature  ( °C )" class="XYGraph (strict)"("Y Scale.Name Label.Text"=w4202) -> ()  [unwired: 2 in, 2 out]
                }
                frame 82 {
                  n3199 = local write "S 84"(w4203) -> ()
                }
                frame 83 {
                  n3200 = local write "S 85"(w4204) -> ()
                }
                frame 84 {
                  n3201 = local write "S 86"(w4205) -> ()
                }
                frame 85 {
                  n3202 = local write "S 87"(w4206) -> ()
                }
                frame 86 {
                  n3203 = local write "S 88"(w4207) -> ()
                }
                frame 87 {
                }
                frame 88 {
                  n3204 = local write "S 90"(w4209) -> ()
                }
                frame 89 {
                  n3205 = local write "S 91"(w4210) -> ()
                }
                frame 90 {
                  n3206 = local write "S 92"(w4211) -> ()
                }
                frame 91 {
                  n3207 = local write "S 93"(w4212) -> ()
                }
                frame 92 {
                  n3208 = local write "S 94"(w4213) -> ()
                }
                frame 93 {
                  n3209 = local write "S 95"(w4214) -> ()
                }
                frame 94 {
                  n3210 = local write "S 96"(w4215) -> ()
                }
                frame 95 {
                  n3211 = local write "S 97"(w4216) -> ()
                }
                frame 96 {
                  n3212 = local write "S 98"(w4217) -> ()
                }
                frame 97 {
                  n3213 = local write "S 99"(w4218) -> ()
                }
                frame 98 {
                  n3214 = local write "S 100"(w4219) -> ()
                }
                frame 99 {
                  n3215 = local write "S 101"(w4220) -> ()
                }
                frame 100 {
                  n3216 = local write "S 102"(w4221) -> ()
                }
                frame 101 {
                  n3217 = local write "S 103"(w4222) -> ()
                }
                frame 102 {
                  n3218 = local write "S 104"(w4223) -> ()
                }
                frame 103 {
                  n3219 = local write "S 105"(w4224) -> ()
                }
                frame 104 {
                  n3220 = local write "S 106"(w4225) -> ()
                }
                frame 105 {
                }
                frame 106 {
                  n3221 = property on="OK Button 17" class="Bool (strict)"("Boolean Text.Text"=w4226) -> ()  [unwired: 2 in, 2 out]
                }
                frame 107 {
                  n3222 = property on="OK Button 16" class="Bool (strict)"("Boolean Text.Text"=w4227) -> ()  [unwired: 2 in, 2 out]
                }
                frame 108 {
                  n3223 = property on="TITTLE" class="Str"("Caption.Text"=w4228) -> ()  [unwired: 2 in, 2 out]
                }
                frame 109 {
                  "String 30" <- w4229
                }
                frame 110 {
                  n3224 = property on="Test Date" class="Str"("Caption.Text"=w4230) -> ()  [unwired: 2 in, 2 out]
                  "String 31" <- w4230
                }
                frame 111 {
                  n3225 = property on="Sample ID" class="Str"("Caption.Text"=w4231) -> ()  [unwired: 2 in, 2 out]
                  "String 32" <- w4231
                }
                frame 112 {
                  n3226 = property on="Tested by" class="Str"("Caption.Text"=w4232) -> ()  [unwired: 2 in, 2 out]
                  "String 33" <- w4232
                }
                frame 113 {
                  n3227 = property on="System Configured Printers 2" class="Arr (strict)"("Caption.Text"=w4233) -> ()  [unwired: 2 in, 2 out]
                }
                frame 114 {
                  n3228 = property on="Selected Printer" class="Str"("Caption.Text"=w4234) -> ()  [unwired: 2 in, 2 out]
                }
                frame 115 {
                  n3229 = property on="Select Printer 3" class="DigNum (strict)"("Caption.Text"=w4235) -> ()  [unwired: 2 in, 2 out]
                }
                frame 116 {
                  n3230 = property on="Print" class="Bool (strict)"("Boolean Text.Text"=w4236) -> ()  [unwired: 2 in, 2 out]
                }
                frame 117 {
                  "String 41" <- w4237
                }
                frame 118 {
                  n3231 = property on="tested by" class="Str"("Caption.Text"=w4238) -> ()  [unwired: 2 in, 2 out]
                }
                frame 119 {
                }
                frame 120 {
                  n3232 = property on="Export" class="Bool (strict)"("Boolean Text.Text"=w4239) -> ()  [unwired: 2 in, 2 out]
                }
                frame 121 {
                }
                frame 122 {
                }
                frame 123 {
                  n3233 = property on="Select File Type" class="Enum (strict)"("Caption.Text"=w4242) -> ()  [unwired: 2 in, 2 out]
                }
                frame 124 {
                  n3234 = property on="s.NO" class="Str"("Caption.Text"=w4243) -> ()  [unwired: 2 in, 2 out]
                  "String 45" <- w4243
                }
                frame 125 {
                  n3235 = property on="trip1 8" class="Bool (strict)"("Boolean Text.Text"=w4244) -> ()  [unwired: 2 in, 2 out]
                }
                frame 126, Default {
                }
              }
            }
          }
          frame #1 {
            w4252 = TRUE ("Visible")
            n3236 = local read "S 91"() -> (w4269:string)
            n3237 = local read "S 90"() -> (w4268:string)
            n3238 = local read "S 88"() -> (w4267:string)
            n3239 = property on="File Path" class="Path"("Caption.Text"=w4268) -> ()  [unwired: 2 in, 2 out]
            n3240 = local read "S 71"() -> (w4262:string)
            n3241 = local read "S 86"() -> (w4264:string)
            n3242 = local read "S 85"() -> (w4265:string)
            n3243 = local read "S 87"() -> (w4263:string)
            n3244 = local read "S 84"() -> (w4266:string)
            n3245 = local read "S 103"() -> (w4251:string)
            n3246 = local read "S 104"() -> (w4250:string)
            n3247 = property on="Password" class="Str"("Caption.Text"=w4265) -> ()  [unwired: 2 in, 2 out]
            n3248 = property on="EDIT" class="Bool (strict)"("Boolean Text.Text"=w4262) -> ()  [unwired: 2 in, 2 out]
            n3249 = property on="SAVE" class="Bool (strict)"("Boolean Text.Text"=w4266) -> ()  [unwired: 2 in, 2 out]
            n3250 = Build Array(w4251, w4250) -> (w4249:string[])
            n3251 = property on="Heater Button" class="Bool (strict)"("Strings [4]"=w4249) -> ()  [unwired: 2 in, 2 out]
            n3252 = local read "S 92"() -> (w4261:string)
            n3253 = local read "S 93"() -> (w4260:string)
            n3254 = local read "S 105"() -> (w4247:string)
            n3255 = local read "S 106"() -> (w4246:string)
            n3256 = Build Array(w4261, w4260) -> ()  [unwired: 1 out]
            n3257 = Build Array(w4247, w4246) -> (w4248:string[])
            n3258 = local read "S 95"() -> (w4258:string)
            n3259 = local read "S 94"() -> (w4259:string)
            n3260 = local read "bs"() -> (w4274:string)
            n3261 = local read "as"() -> (w4275:string)
            n3262 = property on="Humidity" class="Bool (strict)"("Strings [4]"=w4248) -> ()  [unwired: 2 in, 2 out]
            n3263 = Concatenate Strings(w4274, "\r", w4275) -> ()  [unwired: 1 out]
            n3264 = property on="Rh After" class="DigNum (strict)"("Caption.Size to Text?"=TRUE ("Caption.Size to Text")) -> ()  [unwired: 2 in, 2 out]
            n3265 = local read "S 48"() -> (w4298:string)
            n3266 = local read "S 50"() -> (w4296:string)
            n3267 = local read "S 51"() -> (w4295:string)
            n3268 = local read "S 49"() -> (w4297:string)
            n3269 = local read "S 52"() -> (w4294:string)
            n3270 = local read "as"() -> (w4279:string)
            n3271 = local read "bs"() -> (w4280:string)
            n3272 = local read "S 56"() -> (w4293:string)
            n3273 = local read "S 57"() -> (w4292:string)
            n3274 = local read "S 58"() -> (w4291:string)
            n3275 = local read "S 59"() -> (w4290:string)
            n3276 = property on="OPEN" class="Bool (strict)"("Boolean Text.Text"=w4294) -> ()  [unwired: 2 in, 2 out]
            n3277 = property on="OPEN 1" class="Bool (strict)"("Boolean Text.Text"=w4298) -> ()  [unwired: 2 in, 2 out]
            n3278 = property on="OPEN 2" class="Bool (strict)"("Boolean Text.Text"=w4297) -> ()  [unwired: 2 in, 2 out]
            n3279 = property on="OPEN 3" class="Bool (strict)"("Boolean Text.Text"=w4296) -> ()  [unwired: 2 in, 2 out]
            n3280 = property on="OPEN 4" class="Bool (strict)"("Boolean Text.Text"=w4295) -> ()  [unwired: 2 in, 2 out]
            n3281 = Concatenate Strings(w4280, "\r", w4279) -> ()  [unwired: 1 out]
            n3282 = local read "S 102"() -> (w4253:string)
            n3283 = property on="КОФ1" class="DigNum (strict)"("Caption.Text"=w4293) -> ()  [unwired: 2 in, 2 out]
            n3284 = local read "S 98"() -> (w4257:string)
            n3285 = local read "S 99"() -> (w4256:string)
            n3286 = local read "S 100"() -> (w4255:string)
            n3287 = local read "S 101"() -> (w4254:string)
            n3288 = property on="КОФ2" class="DigNum (strict)"("Caption.Text"=w4292) -> ()  [unwired: 2 in, 2 out]
            n3289 = property on="КОФ3" class="DigNum (strict)"("Caption.Text"=w4291) -> ()  [unwired: 2 in, 2 out]
            n3290 = property on="КОФ4" class="DigNum (strict)"("Caption.Text"=w4290) -> ()  [unwired: 2 in, 2 out]
            n3291 = local read "bs"() -> (w4278:string)
            n3292 = local read "as"() -> (w4277:string)
            n3293 = local read "S 60"() -> (w4289:string)
            n3294 = local read "S 54"() -> (w4299:string)
            n3295 = Concatenate Strings(w4278, "\r", w4277) -> ()  [unwired: 1 out]
            n3296 = Concatenate Strings(w4299, w4289) -> ()  [unwired: 1 out]
            n3297 = local read "S 77"() -> (→"String 43":string)
            n3298 = local read "S 76"() -> (w4272:string)
            n3299 = local read "S 78"() -> (w4271:string)
            n3300 = local read "S 71"() -> (w4283:string)
            n3301 = local read "S 66"() -> (w4288:string)
            n3302 = local read "S 67"() -> (w4287:string)
            n3303 = local read "S 68"() -> (w4286:string)
            n3304 = local read "S 69"() -> (w4285:string)
            n3305 = local read "S 70"() -> (w4284:string)
            n3306 = property on="AIR TEMP" class="DigNum (strict)"("Caption.Text"=w4271) -> ()  [unwired: 2 in, 2 out]
            n3307 = property on="Set Strk" class="DigNum (strict)"("Caption.Text"=w4272) -> ()  [unwired: 2 in, 2 out]
            n3308 = property on="SPEED OUT:" class="DigNum (strict)"("Caption.Text"=w4286) -> ()  [unwired: 2 in, 2 out]
            n3309 = property on="EDIT" class="Bool (strict)"("Boolean Text.Text"=w4283) -> ()  [unwired: 2 in, 2 out]
            n3310 = local read "S 79"() -> (w4270:string)
          }
          frame #2 {
          }
        }
        n3311 = local write "Lan flag"(10.0 ("Lan flag")) -> ()
      }
      frame Enabled {
      }
    }
    n3312 = Wait (ms)(milliseconds to wait=u32 2000) -> ()  [unwired: 1 out]
    n3313 = local read "Quit"() -> (w4073:bool)
  }
  n3314 = while {
    shift-right: [w4305] -> _
    shift-left: _ -> [w4306]
    shift-right: [w4303] -> _
    shift-left: T18 {"Read Heave and Surge"="", "Bytes at Heave Port"=0.0, "Heave and Surge COM Port:"="COM9", "Com Port 2"="COM7", "Residual Due"="", "Heave COM Status 2"=TRUE, "Heave COM Status"=TRUE, "Port 2"=TRUE, "Sway PPR"=6400.0, "Surge PPR"=6400.0, "Heave PPR"=6400.0, "Sway Pitch"=2.0, "Surge Pitch"=3.0, "Heave Pitch"=4.0, "Sway Pulses/mm"=320.0, "Surge Pulses/mm"=1600.0, "Heave Pulses/mm"=1600.0, "inner loop"=0.0, "Read Heave and Surge 2"="", "String 36"="", "Write S"=FALSE, "WriteCC1"=[""], "Heave COM Loop"=0, "LastCom"="", "EXIT"=FALSE, "Error Heave"={"status"=TRUE, "code"=-1073807343, "source"=""}} -> [w4302]
    shift-right: [w4300] -> _
    shift-left: enum16{"init", "MAIN", "Panel Close"}."init" -> [w4301]
    stop <- w4304 stop-if-true
    # "HUMIDITY LOOP LOGIC"
    n3315 = case shown="\"MAIN\"" w4301 {
      tunnel: w4306 -> [w4320 w4339 w4394 w4396]
      tunnel: [w4315 w4343 w4394 w4396] -> w4305
      tunnel: [_ _ TRUE _] -> w4304
      tunnel: [w4312 w4341 w4392 w4395] -> w4303
      tunnel: w4302 -> [w4317 w4338 w4392 w4395]
      tunnel: [enum16{"init", "MAIN", "Panel Close"}."MAIN" w4333 _ _] -> w4300
      frame "init" {
        n3316 = local read "C3 :"() -> (w4307:refnum<visa-resource-name>)
        n3317 = Bundle By Name(cluster=w4317, "Heave and Surge COM Port:"=w4307) -> (w4316:T18)
        n3318 = call "Instrument fgv uno.vi"("Enum"=T31."INIT", "error in (no error) 2"=w4320, "INPUT"=w4316) -> ("error"=w4318:errorcluster, "output"=w4314:T18)  [unwired: 6 in, 1 out]
        n3319 = case shown="Error" w4318 {
          selector: w4318 -> [w4322 _]
          tunnel: [w4322 w4326] -> w4315
          tunnel: w4314 -> [w4321 w4324]
          tunnel: [w4321 w4323] -> w4313
          frame No Error {
          }
          frame Error {
            n3320 = call "Instrument fgv uno.vi"("Enum"=T31."ERROR INIT", "INPUT"=w4324) -> ("error"=w4327:errorcluster, "output"=w4323:T18)  [unwired: 7 in, 1 out]
            n3321 = call <vilib>:"Clear Errors.vi"("error in (no error)"=w4327) -> ("error out"=w4326:errorcluster)  [unwired: 5 in, 1 out]
          }
        }
        n3322 = local read "LastCom Humidity"() -> (w4310:string)
        n3323 = Unbundle By Name(w4313) -> ("Heave COM Status 2"=→"COM Status":bool, "Error Heave"=→"Error":errorcluster)  [unwired: 1 out]
        n3324 = Bundle By Name(cluster=w4313, "LastCom"=w4310) -> (w4312:T18)
      }
      frame "MAIN" {
        n3325 = Unbundle By Name(w4338) -> ("Com Port 2"=w4328:refnum<visa-resource-name>)
        n3326 = local read "C3 :"() -> (w4329:refnum<visa-resource-name>)
        n3327 = local write "COM Port Humidity :"(w4328) -> ()
        n3328 = Bundle By Name(cluster=w4338, "Heave and Surge COM Port:"=w4329) -> (w4337:T18)
        n3329 = Equal?(x=w4328, y=w4329) -> (x = y?=w4344:bool)
        n3330 = case shown="True" w4344 {
          tunnel: [w4348 w4365] -> w4343
          tunnel: w4339 -> [w4349 w4371]
          tunnel: w4337 -> [w4347 w4369]
          tunnel: [w4346 w4364] -> w4341
          frame False {
            n3331 = call <vilib>:"Clear Errors.vi"("error in (no error)"=w4349) -> ("error out"=w4345:errorcluster)  [unwired: 5 in, 1 out]
            n3332 = call "Instrument fgv uno.vi"("Enum"=T31."ERROR INIT", "error in (no error) 2"=w4345, "INPUT"=w4347) -> ("error"=w4351:errorcluster, "output"=w4346:T18)  [unwired: 6 in, 1 out]
            n3333 = call <vilib>:"Clear Errors.vi"("error in (no error)"=w4351) -> ("error out"=w4348:errorcluster)  [unwired: 5 in, 1 out]
          }
          frame True {
            n3334 = call "Instrument fgv uno.vi"("Enum"=T31."READ", "error in (no error) 2"=w4371, "INPUT"=w4369) -> ("error"=w4370:errorcluster, "output"=w4363:T18)  [unwired: 6 in, 1 out]
            n3335 = Bundle By Name(cluster=w4363, "String 36"="WRITE HUMIDITY") -> (w4362:T18)
            n3336 = case shown="True" "Write Humidity" {
              selector: "Write Humidity" -> [_ w4391]
              tunnel: w4370 -> [w4384 w4390]
              tunnel: [w4384 w4389] -> w4360
              tunnel: w4362 -> [w4383 w4387]
              tunnel: [w4383 w4386] -> w4359
              frame False {
              }
              frame True {
                n3337 = Not(x=w4391) -> (.not. x?=w4385:bool)
                n3338 = local write "Write Humidity"(w4385) -> ()
                n3339 = call "Instrument fgv uno.vi"("Enum"=T31."MANUAL WRITE", "error in (no error) 2"=w4390, "INPUT"=w4387) -> ("error"=w4389:errorcluster, "output"=w4386:T18)  [unwired: 6 in, 1 out]
              }
            }
            n3340 = Array Size(array="WriteHumidity") -> (size(s)=w4357:i32)
            n3341 = Greater Than 0?(x=w4357) -> (x > 0?=w4356:bool)
            n3342 = call "Instrument fgv uno.vi"("Enum"=T31."WRITE", "error in (no error) 2"=w4360, "WriteCC1"="WriteHumidity", "INPUT"=w4359) -> ("error"=w4367:errorcluster, "WriteCC1 2"=w4358:string[], "output"=w4366:T18)  [unwired: 5 in]
            n3343 = case shown="True" w4356 {
              tunnel: w4358 -> [_ w4373]
              frame False {
              }
              frame True {
                n3344 = local write "WriteHumidity"(w4373) -> ()
              }
            }
            n3345 = case shown="No Error" w4367 {
              selector: w4367 -> [w4374 w4377]
              tunnel: w4366 -> [w4375 w4382]
              tunnel: [w4375 w4381] -> w4364
              tunnel: [w4374 w4379] -> w4365
              frame No Error {
              }
              frame Error {
                n3346 = call <vilib>:"Clear Errors.vi"("error in (no error)"=w4377) -> ("error out"=w4376:errorcluster)  [unwired: 5 in, 1 out]
                n3347 = call "Instrument fgv uno.vi"("Enum"=T31."ERROR INIT", "error in (no error) 2"=w4376, "INPUT"=w4382) -> ("error"=w4380:errorcluster, "output"=w4381:T18)  [unwired: 6 in, 1 out]
                n3348 = call <vilib>:"Clear Errors.vi"("error in (no error)"=w4380) -> ("error out"=w4379:errorcluster)  [unwired: 5 in, 1 out]
              }
            }
            n3349 = Unbundle By Name(w4364) -> ("LastCom"=→"LastCom Humidity":string, "Read Heave and Surge"=→"Read HUMIDITY":string)
          }
        }
        n3350 = Unbundle By Name(w4341) -> ("Heave COM Status 2"=w4342:bool, "Error Heave"=w4330:errorcluster, "Bytes at Heave Port"=→"Bytes at Humidity Port  2":dbl)  [unwired: 1 out]
        n3351 = Unbundle By Name(w4330) -> ("status"=→"Humidity Port":bool)
        n3352 = Not(x=w4342) -> (.not. x?=w4331:bool)
        n3353 = local write "Error"(w4330) -> ()
        n3354 = local read "Quit"() -> (w4334:bool)
        n3355 = local write "COM Status"(w4331) -> ()
